vi "Get voltage range.vi"(8 "error in (no error)":errorcluster, 11 "COM port in":refnum<visa-resource-name>) -> (0 "error out":errorcluster, 2 "Voltage range":i32, 3 "COM port out":refnum<visa-resource-name>)   [LabVIEW 2020]
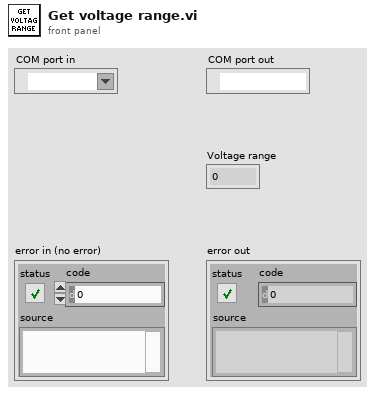
[diagram p1: front panel]
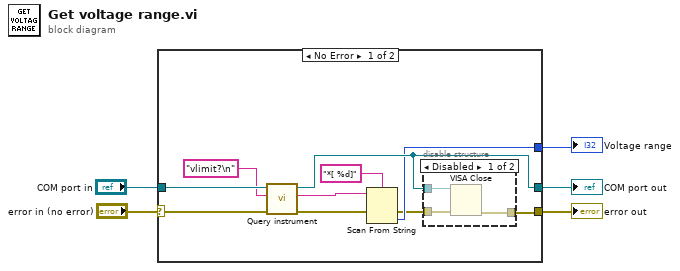
[diagram p0: block diagram]
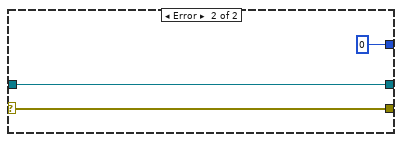
[diagram p3: hidden frame]
diagram:
  n1 = case shown="No Error" "error in (no error)" {
    selector: "error in (no error)" -> [w15 w22]
    tunnel: [w12 w22] -> w4
    tunnel: "COM port in" -> [w14 w21]
    tunnel: [w11 w21] -> w2
    tunnel: [w8 0] -> w1
    frame No Error {
      n2 = call "Query instrument.vi"("error in (no error)"=w15, "Command"="vlimit?\n", "COM port in"=w14) -> ("error out"=w7:errorcluster, "read buffer"=w10:string, "COM port out"=w11:refnum<visa-resource-name>)  [unwired: 6 in]
      n3 = Scan From String(format string="*[ %d]", input string=w10, error in=w7) -> (error out=w6:errorcluster, output 1=w8:i32)  [unwired: 2 in, 2 out]
      n4 = disable-structure shown="Disabled" {
        disable-tunnel: [w18 w19] -> w12
        disable-tunnel: w11 -> [w17 _]
        disable-tunnel: w6 -> [w16 w19]
        frame Disabled {
          n5 = VISA Close(VISA resource name=w17, error in (no error)=w16) -> (error out=w18:errorcluster)
        }
        frame Enabled {
        }
      }
    }
    frame Error {
    }
  }
  "error out" <- w4
  "COM port out" <- w2
  "Voltage range" <- w1
